vi "Modules - Explorer.vi"(8 "error in":errorcluster) -> (0 "error out":errorcluster)   [LabVIEW 2019]
uses:
  Controls/Explorer - State.ctl
  Controls/eFGV States.ctl
  Controls/Explorer - Data Structure.ctl
  <vilib>/httpClient/ClientHandle.ctl
  Controls/FGV States.ctl
  Controls/JSON - Fileid.ctl
  <vilib>/httpClient/POSTBuffer.vi
  <vilib>/httpClient/LabVIEWHTTPClient.lvlib
panel:
  in  "Pin":bool
  in  "Refresh":bool
  in  "Tab":enum32{"Running", "Archive"}(radio)
  in  "TreeDone":string(tree)
  in  "TreeRun":string(tree)
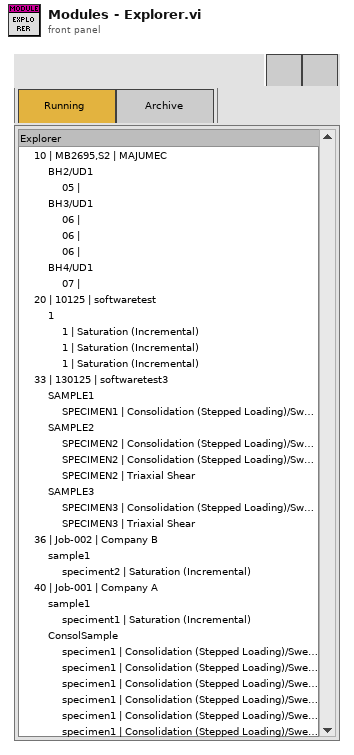
[diagram p1: front panel]
types:
  T1 = typedef "Explorer - State.ctl" = enum16{"Init", "Idle", "DoubleClick", "GetInfo", "Porpulate", "Sort", "Prepare to Load", "Load", "Close", "Exit"}
  T2 = enum32{"invalid app kind", "Development System", "Run Time System", "Student Edition", "Embedded LabVIEW", "Evaluation", "Custom"}
  T3 = typedef "Explorer - Data Structure.ctl" = cluster{"Ref":T4, "TestData":string, "TestNameRun":string[], "TestNameDone":string[], "Selected Tag":string, "Selected Index":i32, "LoadRun?":bool, "NameRun":string[], "NameDone":string[], "fileid":string[], "testname":string[]}
  T4 = typedef "LabVIEWHTTPClient.lvlib/ClientHandle.ctl" = refnum<k1>
  T5 = typedef "eFGV States.ctl" = enum16{"Init", "Read", "Write", "Exit"}
  T6 = enum32{"Invalid", "Standard", "Closed", "Hidden", "Minimized", "Maximized"}
  T7 = typedef "FGV States.ctl" = enum16{"Read", "Write"}
  T8 = typedef "JSON - Fileid.ctl" = cluster{"status":string, "data":cluster{"id":string, "created_date":string, "testname":string, "jobno":string, "jobdesc":string, "sampleid":string, "date":string, "specimentno":string, "depth":string, "height":string, "diameter":string, "weight":string, "done":string}[]}
  T9 = cluster{"RunTest":refnum<vi>, "Name":string, "FileId":string, "Status":string}
  T10 = cluster{"id":string, "created_date":string, "testname":string, "jobno":string, "jobdesc":string, "sampleid":string, "date":string, "specimentno":string, "depth":string, "height":string, "diameter":string, "weight":string, "done":string}[]
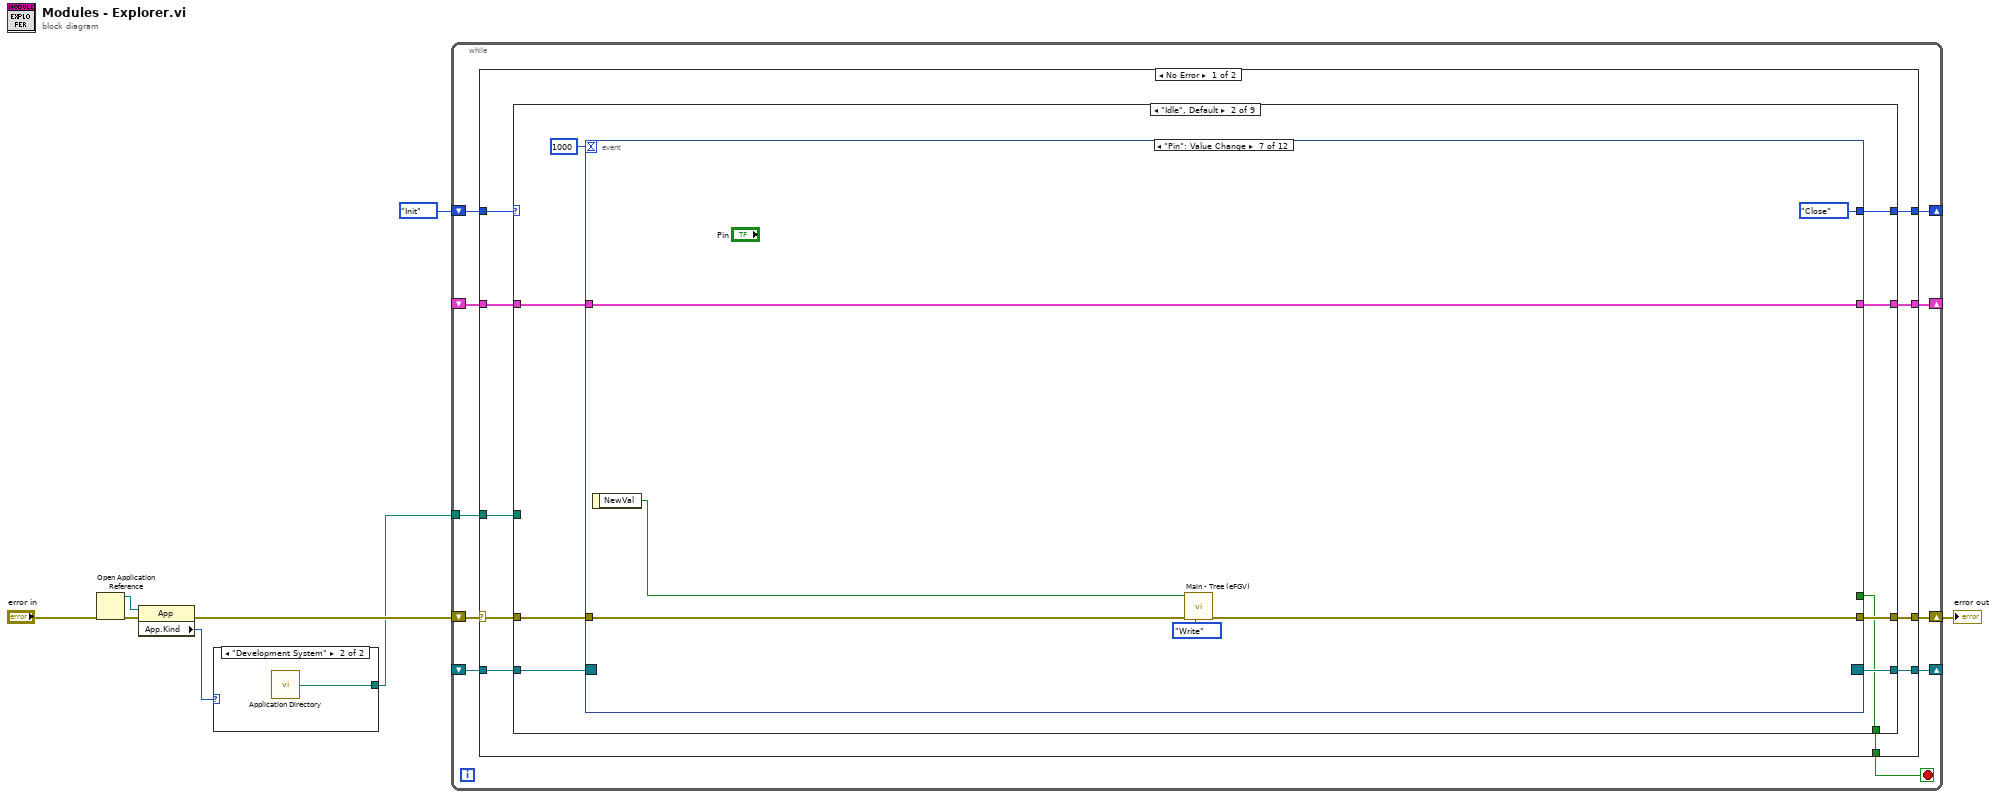
[diagram p0: block diagram]
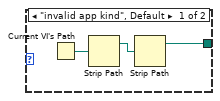
[diagram p2: hidden frame]
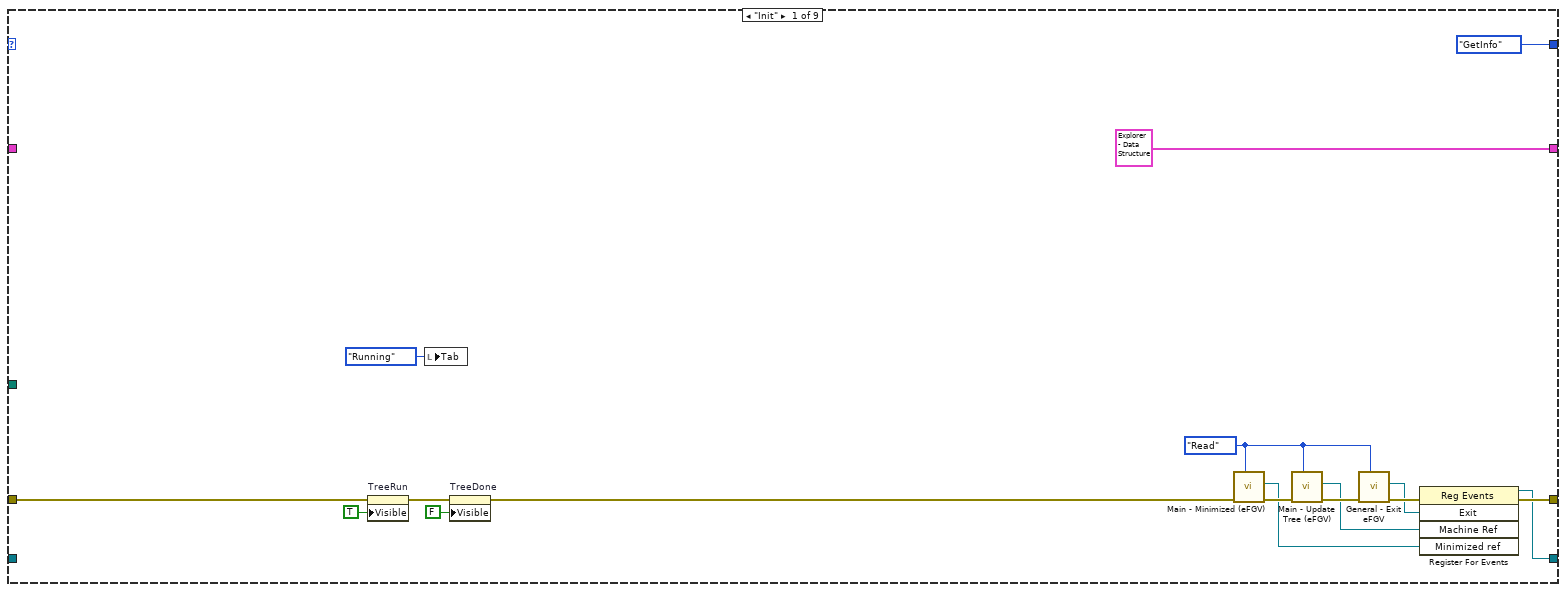
[diagram p3: hidden frame]
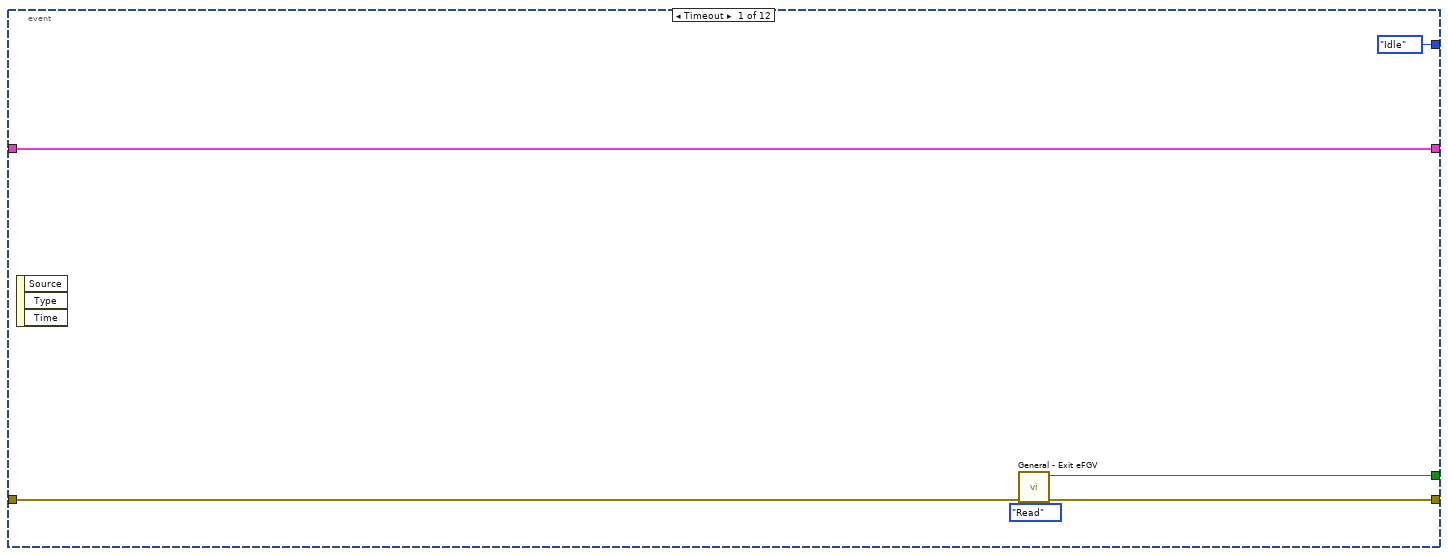
[diagram p4: hidden frame]
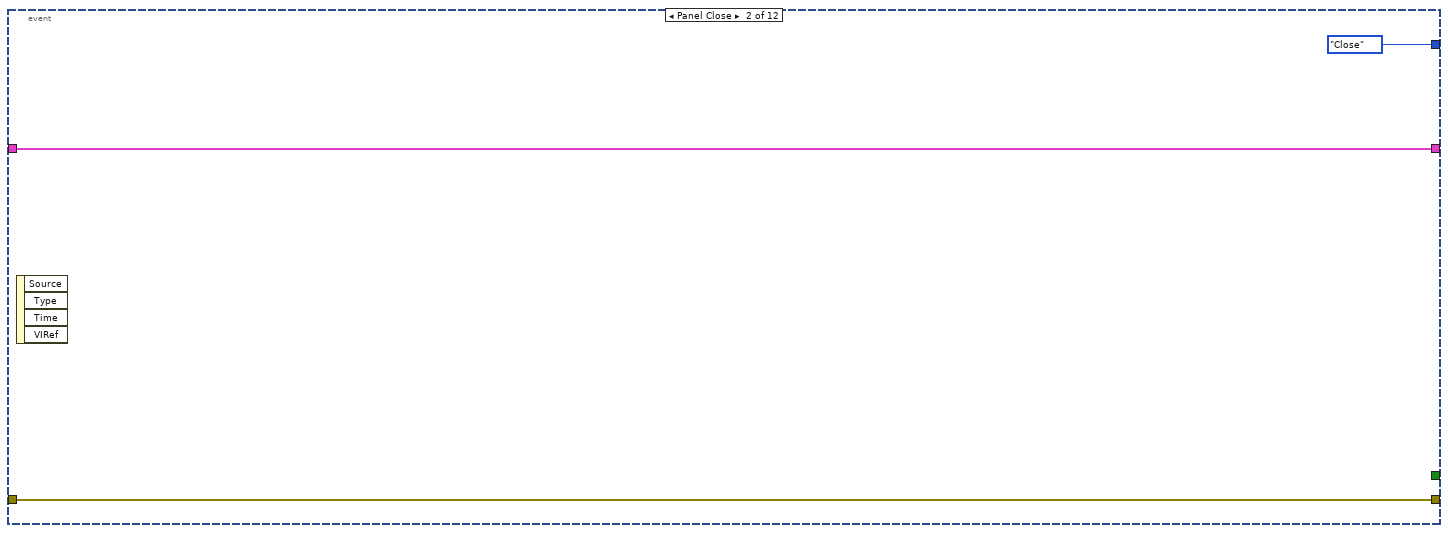
[diagram p5: hidden frame]
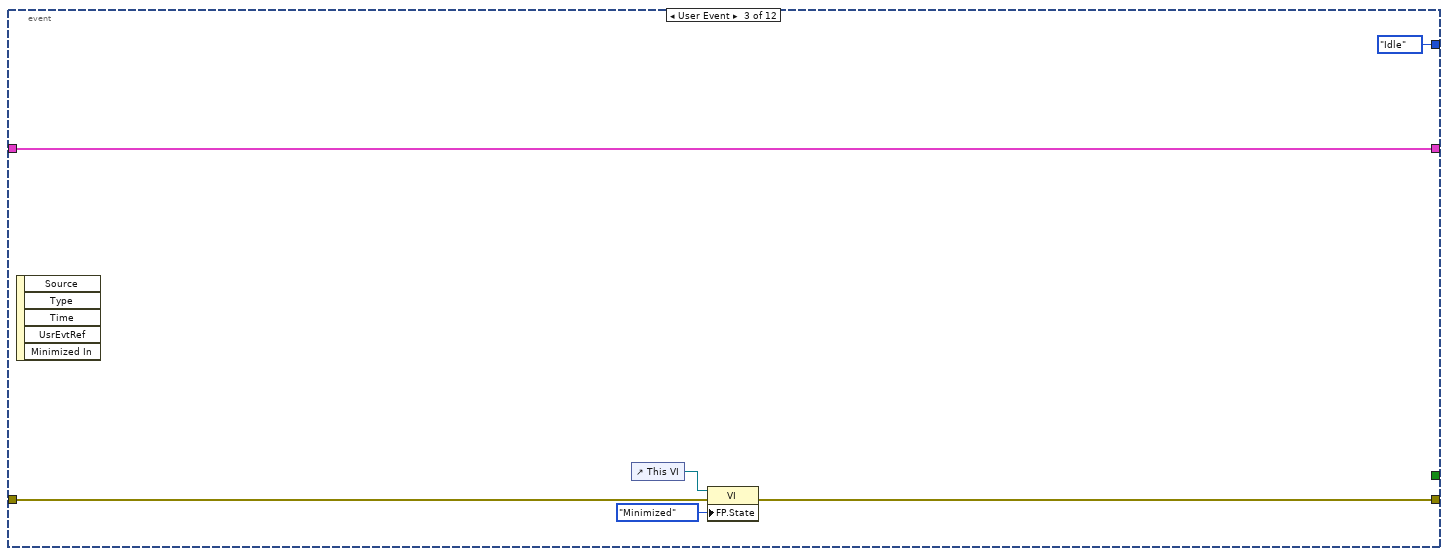
[diagram p6: hidden frame]
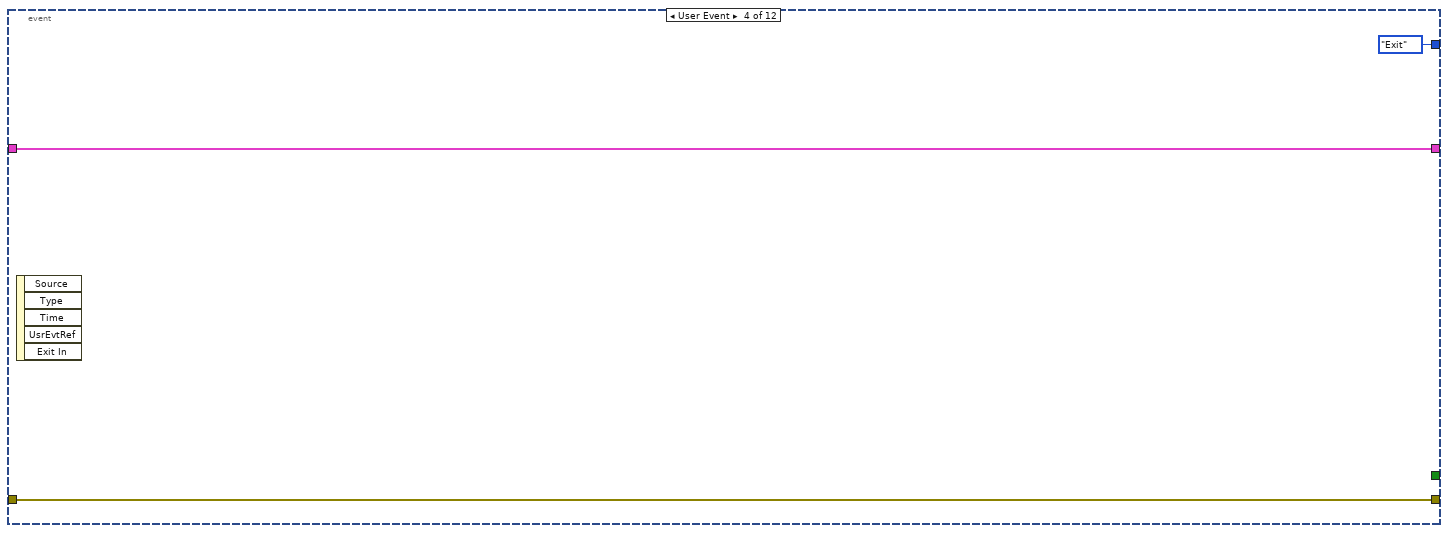
[diagram p7: hidden frame]
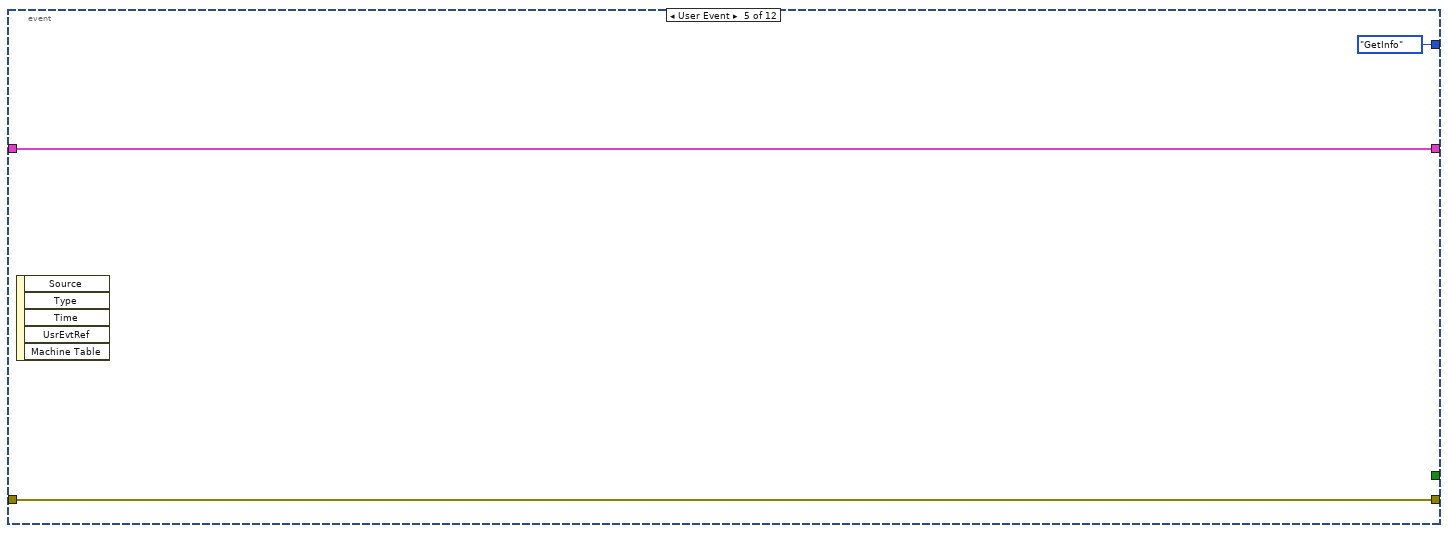
[diagram p8: hidden frame]
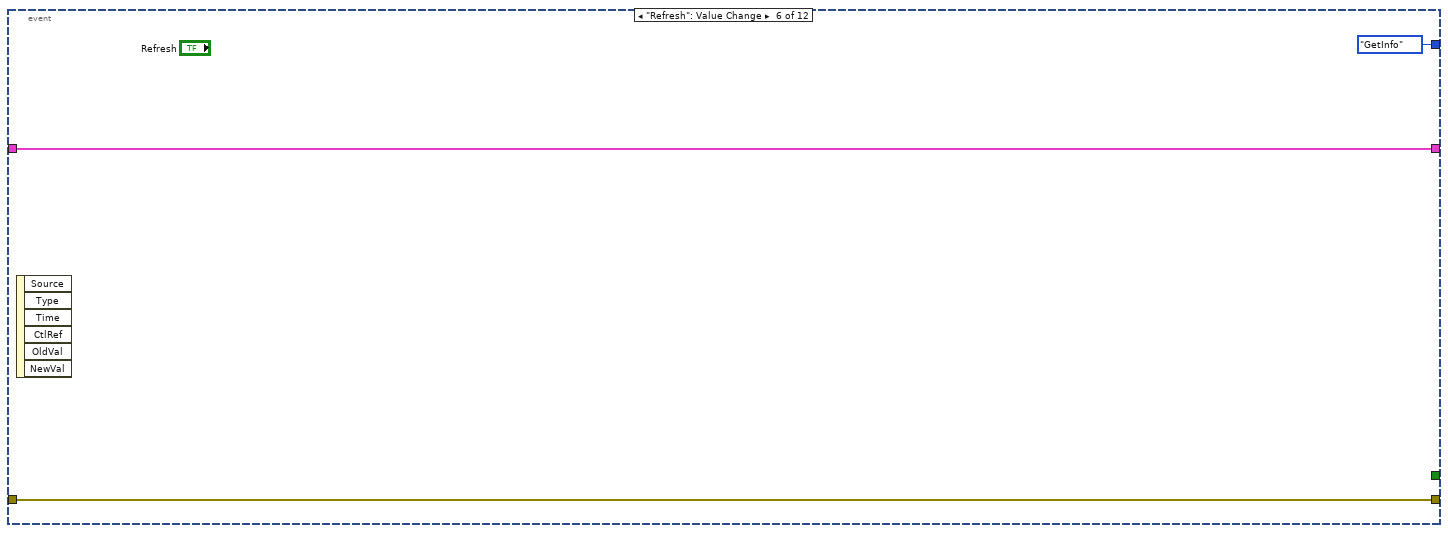
[diagram p9: hidden frame]
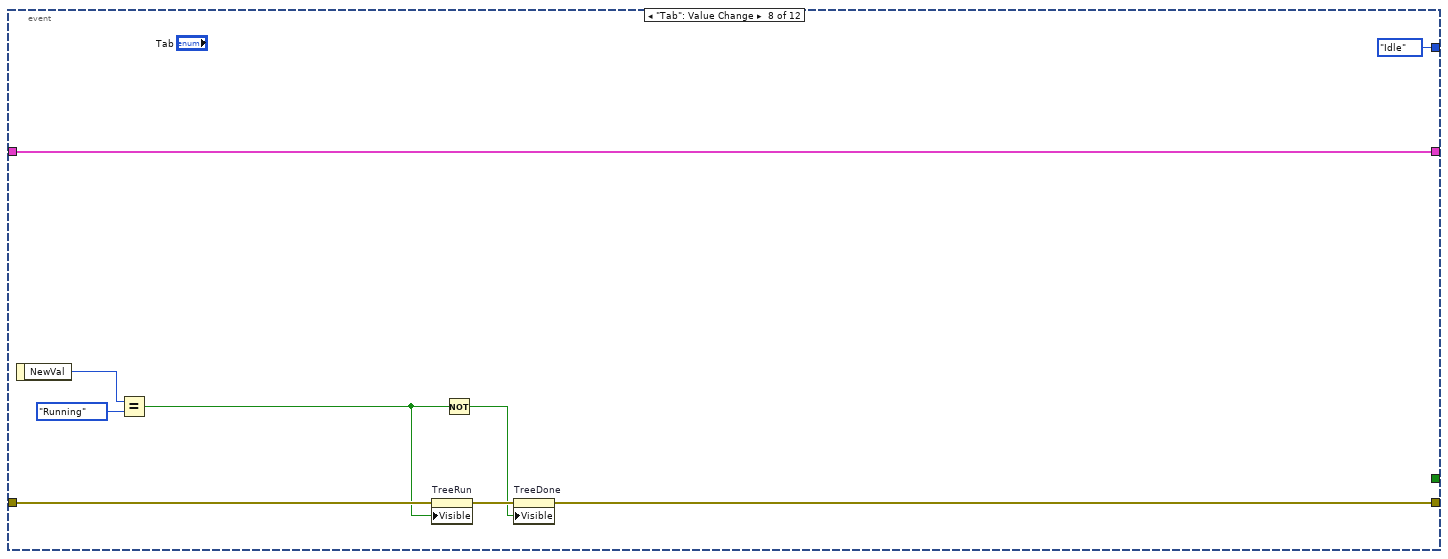
[diagram p10: hidden frame]
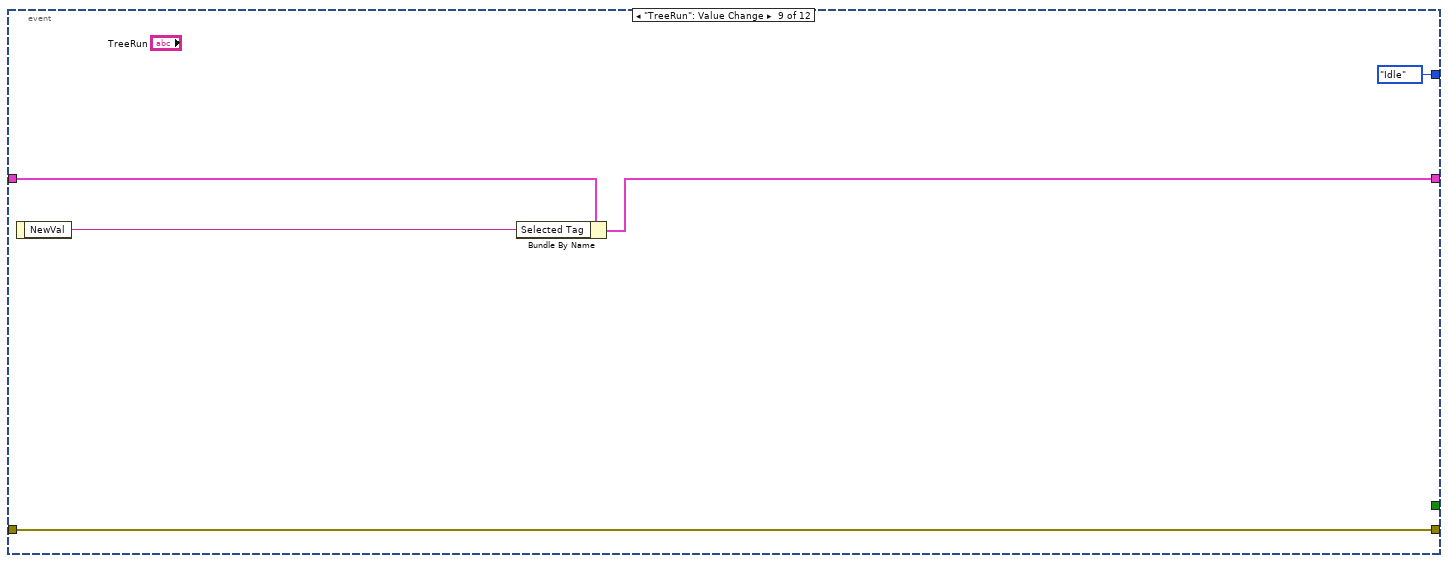
[diagram p11: hidden frame]
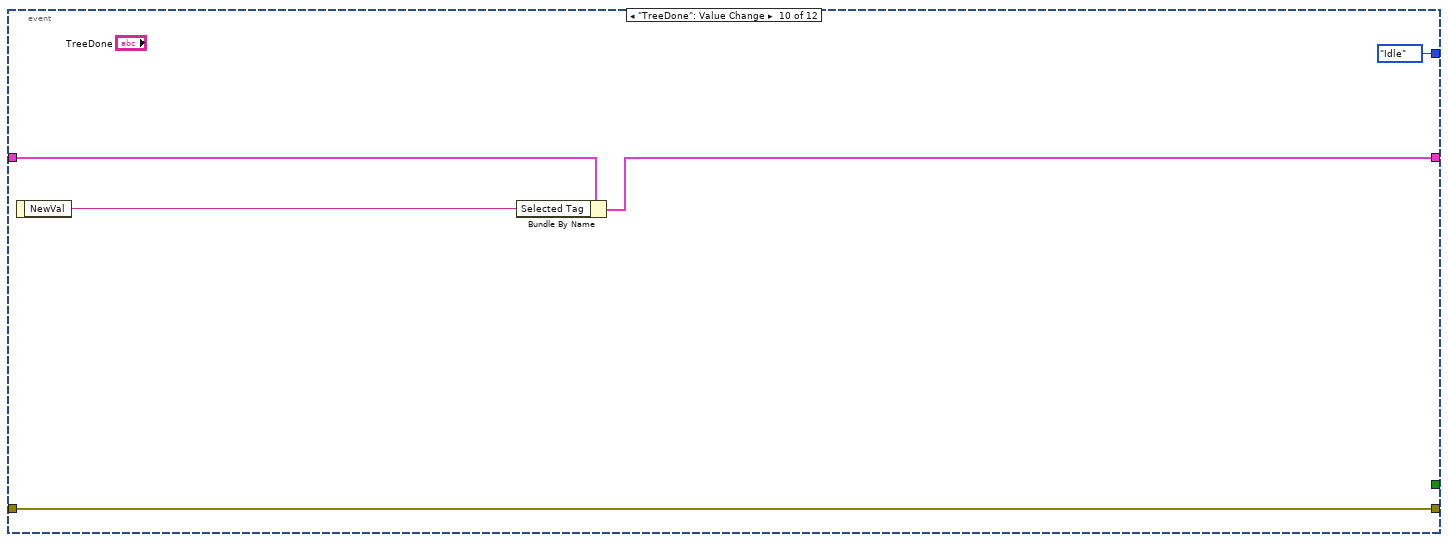
[diagram p12: hidden frame]
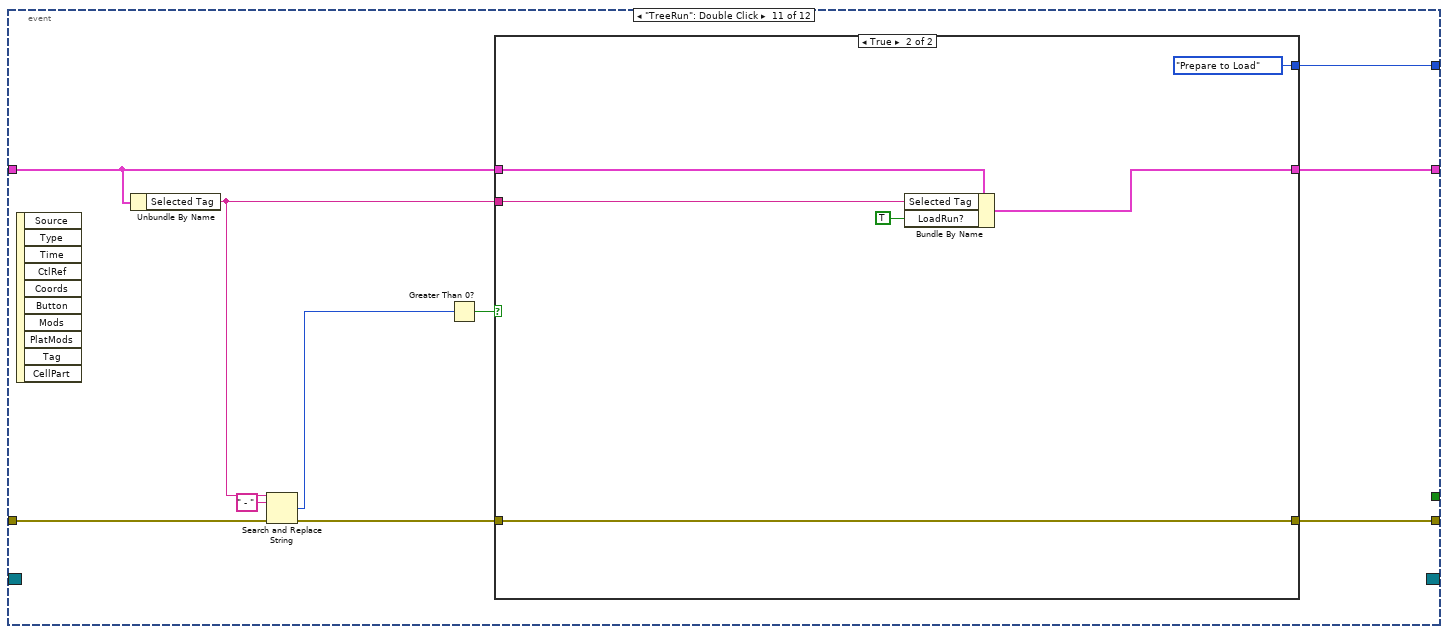
[diagram p13: hidden frame]
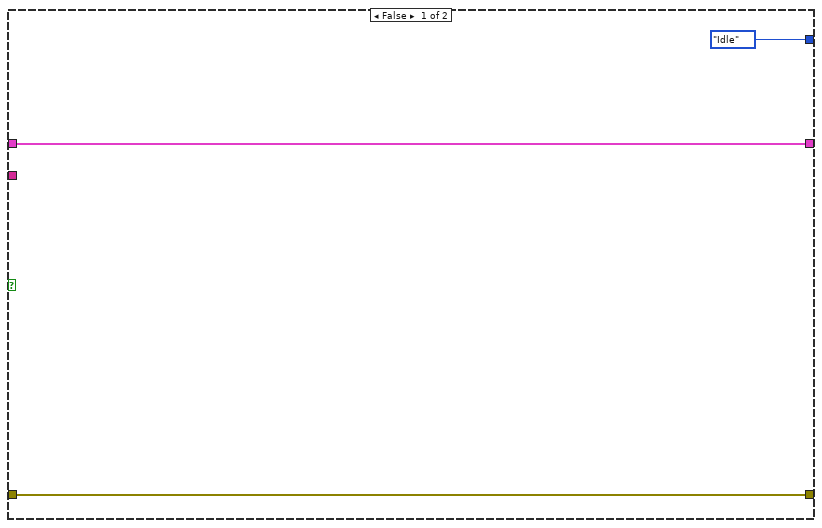
[diagram p14: hidden frame]
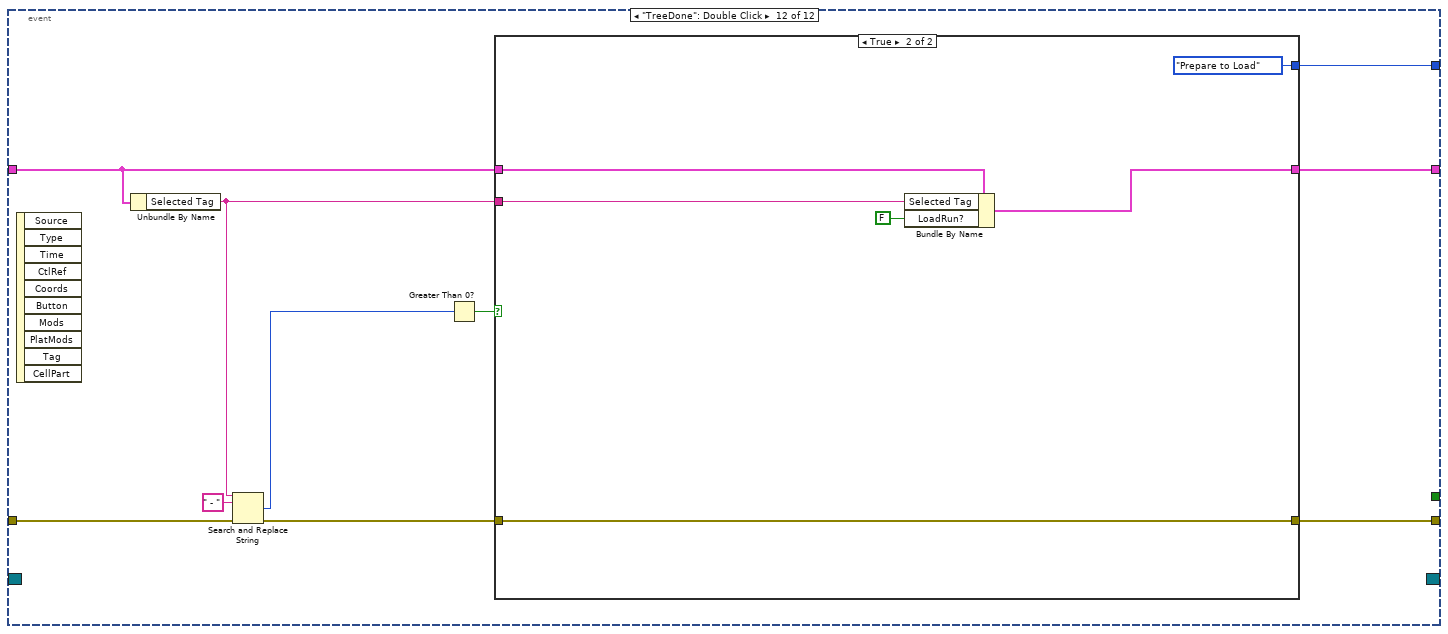
[diagram p15: hidden frame]
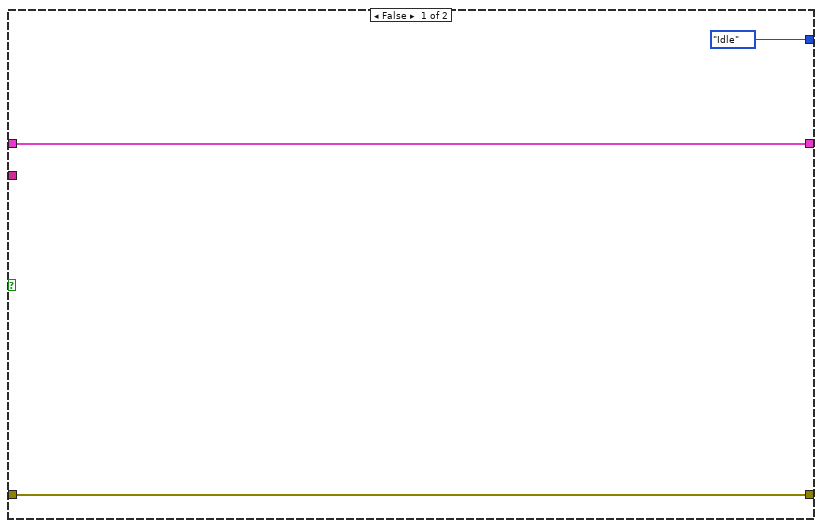
[diagram p16: hidden frame]
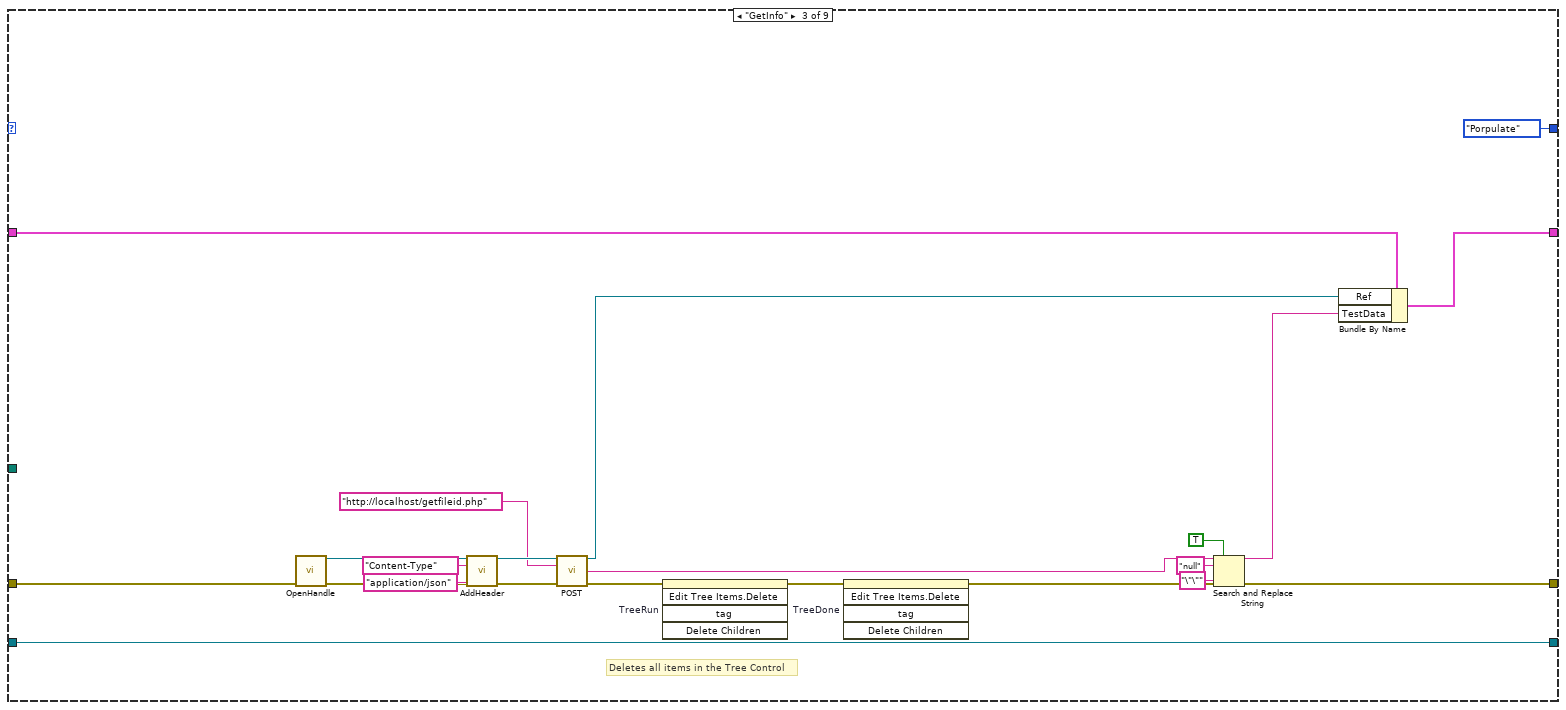
[diagram p17: hidden frame]
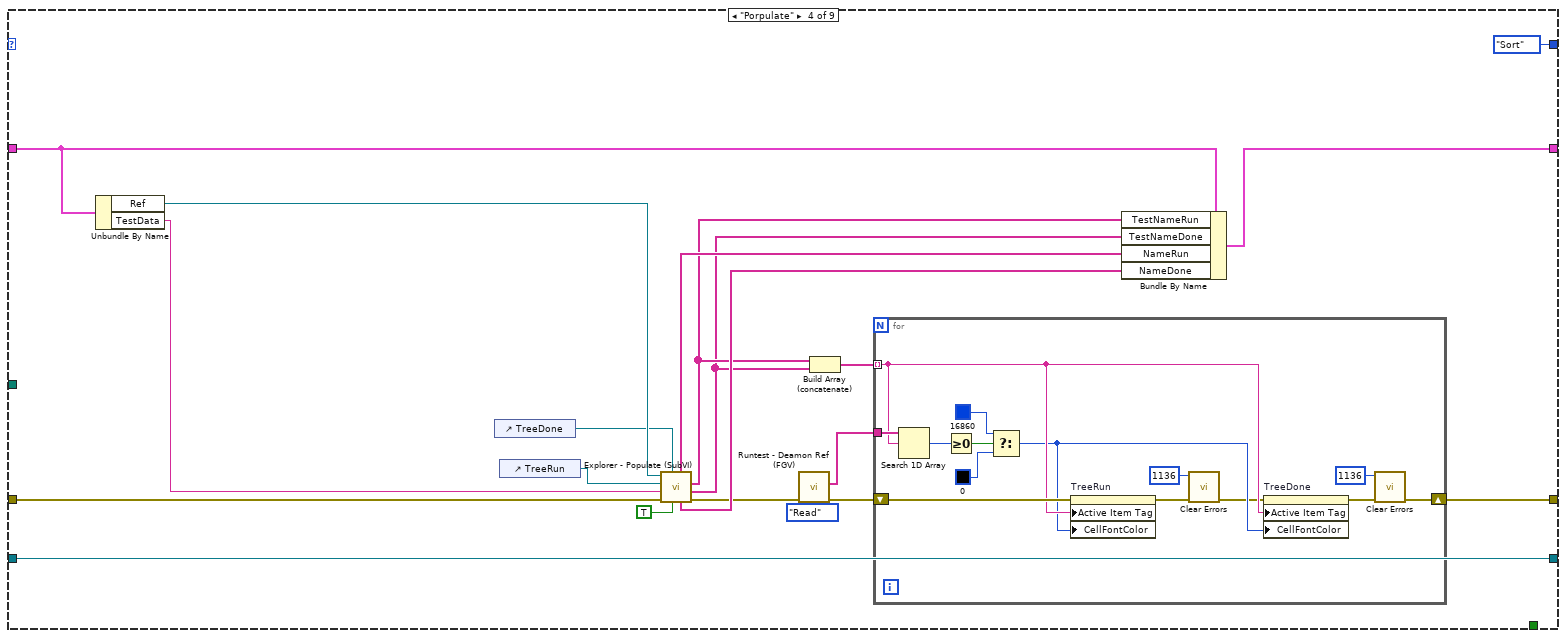
[diagram p18: hidden frame]
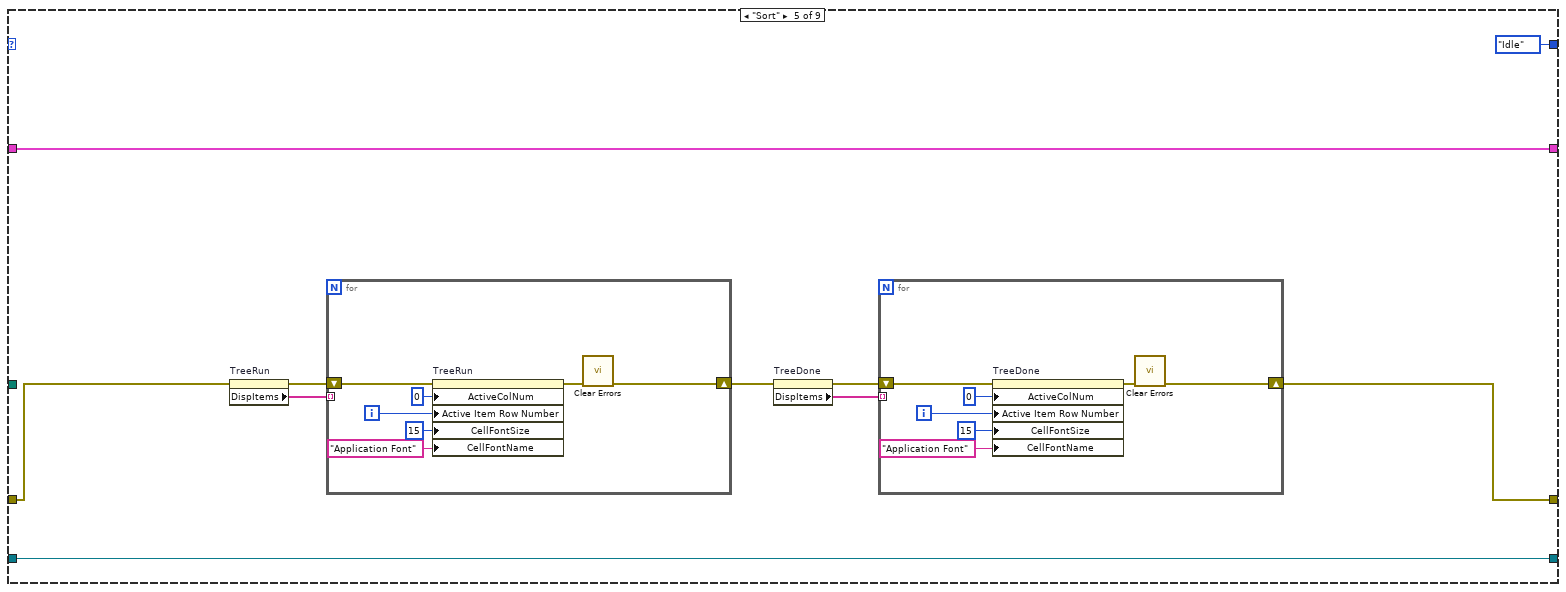
[diagram p19: hidden frame]
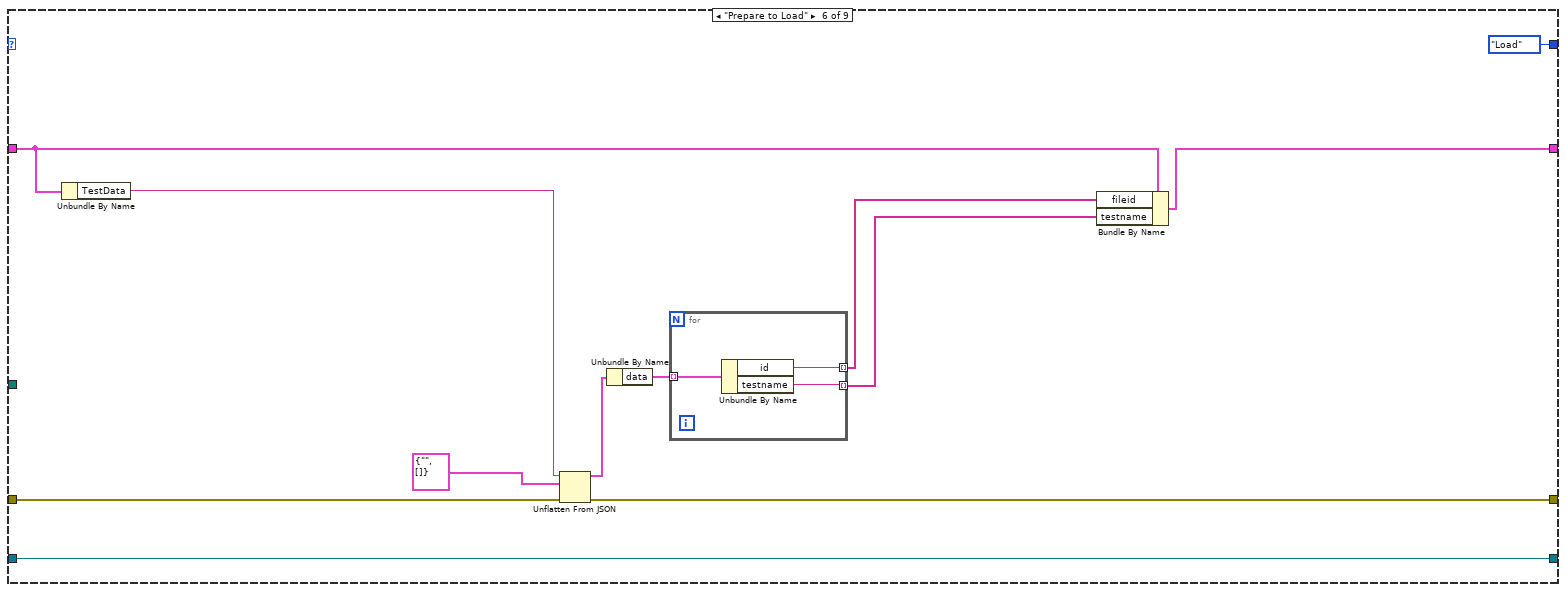
[diagram p20: hidden frame]
diagram:
  n1 = Open Application Reference(8:"error in") -> (0:w6:errorcluster, 3:w5:refnum<vi>)  [unwired: 3 in]
  n2 = property class="App"(reference=w5, error in=w6) -> (error out=w2:errorcluster, "App.Kind"=w4:T2)  [unwired: 1 out]
  n3 = case shown="\"Development System\"" w4 {
    tunnel: [w9 w12] -> w1
    frame "invalid app kind", Default {
      n4 = Current VI's Path() -> (path=w11:path)
      n5 = Strip Path(path=w11) -> (stripped path=w10:path)  [unwired: 1 out]
      n6 = Strip Path(path=w10) -> (stripped path=w9:path)  [unwired: 1 out]
    }
    frame "Development System" {
      n7 = call <vilib>:"Application Directory.vi"() -> ("Application Directory"=w12:path)
    }
  }
  n8 = while {
    shift-right: [w21] -> w8
    shift-left: w2 -> [w22]
    shift-right: [w19] -> _
    shift-left: _ -> [w18]
    shift-right: [w16] -> _
    shift-left: Explorer_-_State."Init" ("Enum") -> [w17]
    shift-right: [w15] -> _
    shift-left: _ -> [w14]
    tunnel: w1 -> [w13]
    stop <- w20 stop-if-true
    n9 = case shown="No Error" w22 {
      selector: w22 -> [w32 w433]
      tunnel: [w31 w432] -> w21
      tunnel: [w30 _] -> w20
      tunnel: [w29 w430] -> w19
      tunnel: w18 -> [w28 w430]
      tunnel: w17 -> [w27 _]
      tunnel: [w26 Explorer_-_State."Idle" ("Enum")] -> w16
      tunnel: [w25 w429] -> w15
      tunnel: w14 -> [w24 w429]
      tunnel: w13 -> [w23 _]
      frame No Error {
        n10 = case shown="\"Idle\", Default" w27 {
          tunnel: w32 -> [w38 w57 w151 w185 w207 w234 w246 w418 w426]
          tunnel: [w47 w58 w150 w168 w202 w235 w247 w417 w426] -> w31
          tunnel: [_ w50 _ _ _ _ _ _ TRUE] -> w30
          tunnel: [w46 w55 w167 w187 w211 w237 w248 w422 w423] -> w29
          tunnel: w28 -> [_ w56 w167 w187 w211 w237 w248 w422 w423]
          tunnel: [Explorer_-_State."GetInfo" ("Enum") w54 Explorer_-_State."Porpulate" ("Enum") Explorer_-_State."Sort" ("Enum") Explorer_-_State."Idle" ("Enum") Explorer_-_State."Load" ("Enum") Explorer_-_State."Idle" ("Enum") Explorer_-_State."Idle" ("Enum") Explorer_-_State."Exit" ("Enum")] -> w26
          tunnel: [T3 {"Ref"=refnum, "TestData"="", "TestNameRun"=[], "TestNameDone"=[], "Selected Tag"="", "Selected Index"=0, "LoadRun?"=FALSE, "NameRun"=[], "NameDone"=[], "fileid"=[], "testname"=[]} w53 w149 w181 w208 w227 w243 w421 w424] -> w25
          tunnel: w24 -> [_ w52 w148 w180 w208 w226 w242 w421 w424]
          tunnel: w23 -> [_ _ _ _ _ _ w241 _ _]
          frame "Init" {
            w33 = eFGV_States."Read" ("eFGV States")
            n11 = property on="TreeRun" class="Tree (strict)"(error in=w38, "Visible"=TRUE) -> (error out=w39:errorcluster)  [unwired: 1 in, 1 out]
            n12 = local write "Tab"(enum32{"Running", "Archive"}."Running" ("Tab")) -> ()
            n13 = property on="TreeDone" class="Tree (strict)"(error in=w39, "Visible"=FALSE) -> (error out=w36:errorcluster)  [unwired: 1 in, 1 out]
            n14 = call "Main - Minimized (eFGV).vi"("Action"=w33, "error in"=w36) -> ("error out"=w35:errorcluster, "Minimized ref"=w34:refnum<user-event>)  [unwired: 7 in, 1 out]
            n15 = call "Main - Update Tree (eFGV).vi"("Action"=w33, "error in"=w35) -> ("error out"=w43:errorcluster, "Machine Ref"=w42:refnum<user-event>)  [unwired: 7 in, 1 out]
            n16 = call "General - Exit eFGV.vi"("eFGV States"=w33, "error in (no error)"=w43) -> ("error out"=w49:errorcluster, "Exit"=w48:refnum<user-event>)  [unwired: 7 in, 1 out]
            n17 = register-events(error in=w49, w48, w42, w34) -> (reference out=w46:refnum<event-registration>, error out=w47:errorcluster)  [unwired: 1 in]
          }
          frame "Idle", Default {
            n18 = event shown="[6] \"Pin\": Value Change" {
              selector: w56 -> [_ _ _ _ _ _ _ _ _ _ _ _]
              dyn-events: [_ _ _ _ _ _ _ _ _ _ _ _] -> w55
              timeout: 1000 -> [_ _ _ _ _ _ _ _ _ _ _ _]
              tunnel: w57 -> [w60 w67 w68 w76 w79 w82 w85 w93 w101 w106 w111 w130]
              tunnel: [w61 w67 w69 w76 w79 w82 w86 w94 w101 w106 w116 w135] -> w58
              tunnel: [Explorer_-_State."Idle" ("Enum") Explorer_-_State."Close" ("Enum") Explorer_-_State."Idle" ("Enum") Explorer_-_State."Exit" ("Enum") Explorer_-_State."GetInfo" ("Enum") Explorer_-_State."GetInfo" ("Enum") Explorer_-_State."Close" ("Enum") Explorer_-_State."Idle" ("Enum") Explorer_-_State."Idle" ("Enum") Explorer_-_State."Idle" ("Enum") w113 w132] -> w54
              tunnel: [w63 w65 w73 w75 w78 w81 w88 w97 w100 w105 w114 w133] -> w53
              tunnel: w52 -> [w63 w65 w73 w75 w78 w81 w88 w97 w99 w104 w115 w134]
              tunnel: [w59 _ _ _ _ _ _ _ _ _ _ _] -> w50
              event Timeout {
                n19 = event-data() -> ()  [unwired: 1 in, 3 out]
                n20 = call "General - Exit eFGV.vi"("eFGV States"=eFGV_States."Read", "error in (no error)"=w60) -> ("error out"=w61:errorcluster, "Exit Out"=w59:bool)  [unwired: 7 in, 1 out]
              }
              event Panel Close {
                n21 = event-data() -> ()  [unwired: 1 in, 4 out]
              }
              event User Event {
                n22 = event-data() -> ()  [unwired: 1 in, 5 out]
                n23 = control-ref of="This VI"() -> (w71:refnum<vi>)
                n24 = property class="VI"(reference=w71, error in=w68, "FP.State"=T6."Minimized" ("Front Panel Window:State")) -> (error out=w69:errorcluster)  [unwired: 1 out]
              }
              event User Event {
                n25 = event-data() -> ()  [unwired: 1 in, 5 out]
              }
              event User Event {
                n26 = event-data() -> ()  [unwired: 1 in, 5 out]
              }
              event "Refresh": Value Change {
                n27 = event-data() -> ()  [unwired: 1 in, 6 out]
              }
              event "Pin": Value Change {
                n28 = event-data() -> ("NewVal"=w84:bool)  [unwired: 1 in]
                n29 = call "Main - Tree (eFGV).vi"("Action"=eFGV_States."Write", "error in"=w85, "Pin"=w84) -> ("error out"=w86:errorcluster)  [unwired: 6 in, 2 out]
              }
              event "Tab": Value Change {
                n30 = event-data() -> ("NewVal"=w92:enum32{"Running", "Archive"})  [unwired: 1 in]
                n31 = Equal?(x=w92, y=enum32{"Running", "Archive"}."Running") -> (x = y?=w90:bool)
                n32 = property on="TreeRun" class="Tree (strict)"(error in=w93, "Visible"=w90) -> (error out=w95:errorcluster)  [unwired: 1 in, 1 out]
                n33 = Not(x=w90) -> (.not. x?=w89:bool)
                n34 = property on="TreeDone" class="Tree (strict)"(error in=w95, "Visible"=w89) -> (error out=w94:errorcluster)  [unwired: 1 in, 1 out]
              }
              event "TreeRun": Value Change {
                n35 = event-data() -> ("NewVal"=w98:string)  [unwired: 1 in]
                n36 = Bundle By Name(cluster=w99, "Selected Tag"=w98) -> (w100:T3)
              }
              event "TreeDone": Value Change {
                n37 = event-data() -> ("NewVal"=w103:string)  [unwired: 1 in]
                n38 = Bundle By Name(cluster=w104, "Selected Tag"=w103) -> (w105:T3)
              }
              event "TreeRun": Double Click {
                n39 = event-data() -> ()  [unwired: 1 in, 10 out]
                n40 = Unbundle By Name(w115) -> ("Selected Tag"=w110:string)
                n41 = Search and Replace String(input string=w110, search string=" - ", error in=w111) -> (number of replacements=w108:i32, error out=w112:errorcluster)  [unwired: 5 in, 2 out]
                n42 = Greater Than 0?(x=w108) -> (x > 0?=w117:bool)
                n43 = case shown="True" w117 {
                  tunnel: w112 -> [w120 w122]
                  tunnel: [w120 w122] -> w116
                  tunnel: w115 -> [w119 w126]
                  tunnel: [w119 w125] -> w114
                  tunnel: w110 -> [_ w121]
                  tunnel: [Explorer_-_State."Idle" ("Enum") Explorer_-_State."Prepare to Load" ("Enum")] -> w113
                  frame False {
                  }
                  frame True {
                    n44 = Bundle By Name(cluster=w126, "Selected Tag"=w121, "LoadRun?"=TRUE) -> (w125:T3)
                  }
                }
              }
              event "TreeDone": Double Click {
                n45 = event-data() -> ()  [unwired: 1 in, 10 out]
                n46 = Unbundle By Name(w134) -> ("Selected Tag"=w129:string)
                n47 = Search and Replace String(input string=w129, search string=" - ", error in=w130) -> (number of replacements=w127:i32, error out=w131:errorcluster)  [unwired: 5 in, 2 out]
                n48 = Greater Than 0?(x=w127) -> (x > 0?=w136:bool)
                n49 = case shown="True" w136 {
                  tunnel: w131 -> [w139 w141]
                  tunnel: [w139 w141] -> w135
                  tunnel: w134 -> [w138 w145]
                  tunnel: [w138 w144] -> w133
                  tunnel: w129 -> [_ w140]
                  tunnel: [Explorer_-_State."Idle" ("Enum") Explorer_-_State."Prepare to Load" ("Enum")] -> w132
                  frame False {
                  }
                  frame True {
                    n50 = Bundle By Name(cluster=w145, "Selected Tag"=w140, "LoadRun?"=FALSE) -> (w144:T3)
                  }
                }
              }
            }
          }
          frame "GetInfo" {
            # "Deletes all items in the Tree Control"
            n51 = call <vilib>:"OpenHandle.vi"("error in (no error)"=w151) -> ("client handle out"=w162:T4, "error out"=w160:errorcluster)  [unwired: 13 in]
            n52 = call <vilib>:"AddHeader.vi"("client handle"=w162, "header"="Content-Type", "value"="application/json", "error in (no error)"=w160) -> ("client handle out"=w163:T4, "error out"=w161:errorcluster)  [unwired: 10 in]
            n53 = call-poly <vilib>:"POST.vi"("client handle"=w163, "url"="http://localhost/getfileid.php", "error in (no error)"=w161) -> ("client handle out"=w153:T4, "body"=w156:string, "error out"=w158:errorcluster)  [unwired: 9 in, 1 out]
            n54 = invoke on="TreeRun" class="Tree (strict)" method="Edit Tree Items.Delete"(error in=w158) -> (error out=w147:errorcluster)  [unwired: 4 in, 4 out]
            n55 = invoke on="TreeDone" class="Tree (strict)" method="Edit Tree Items.Delete"(error in=w147) -> (error out=w146:errorcluster)  [unwired: 4 in, 4 out]
            n56 = Search and Replace String(replace all?=TRUE ("replace all? (F)"), input string=w156, search string="null", replace string="\"\"" ("replace string (\"\")"), error in=w146) -> (result string=w152:string, error out=w150:errorcluster)  [unwired: 3 in, 2 out]
            n57 = Bundle By Name(cluster=w148, "Ref"=w153, "TestData"=w152) -> (w149:T3)
          }
          frame "Porpulate" {
            n58 = Unbundle By Name(w180) -> ("Ref"=w183:T4, "TestData"=w184:string)
            n59 = control-ref of="TreeDone"() -> (w179:refnum<vi>)
            n60 = control-ref of="TreeRun"() -> (w182:refnum<vi>)
            n61 = call "Explorer - Populate (SubVI).vi"("Asc?"=TRUE, "TreeDone"=w179, "error in (no error)"=w185, "Test Data"=w184, "TreeRun"=w182, "RefIn"=w183) -> ("error out"=w174:errorcluster, "TestName Done"=w171:string[], "TestName Running"=w172:string[], "Name Done"=w176:string[], "Name Running"=w177:string[])  [unwired: 1 out]
            n62 = call "Runtest - Deamon Ref (FGV).vi"("Action"=FGV_States."Read", "error in"=w174) -> ("error out"=w169:errorcluster, "Name out"=w173:string[])  [unwired: 7 in, 1 out]
            n63 = Build Array (concatenate)(w172, w171) -> (w170:string[])
            n64 = for {
              tunnel: w173 -> [w201]
              tunnel: w170 -> [w193] mode=indexing
              shift-right: [w189] -> w168
              shift-left: w169 -> [w196]
              n65 = Search 1D Array(1D array=w201, element=w193) -> (index of element=w200:i32)  [unwired: 1 in]
              n66 = Greater Or Equal To 0?(x=w200) -> (x >= 0?=w199:bool)
              n67 = Select(t=u32 16860 ("Active Cell:Cell Font:Color"), s=w199, f=u32 0 ("Active Cell:Cell Font:Color")) -> (s? t:f=w192:u32)
              n68 = property on="TreeRun" class="Tree (strict)"(error in=w196, "Active Item Tag"=w193, "CellFontColor"=w192) -> (error out=w195:errorcluster)  [unwired: 1 in, 1 out]
              n69 = call <vilib>:"Clear Errors.vi"("error in (no error)"=w195, "specific error code to clear (0: all)"=1136) -> ("error out"=w191:errorcluster)  [unwired: 4 in, 1 out]
              n70 = property on="TreeDone" class="Tree (strict)"(error in=w191, "Active Item Tag"=w193, "CellFontColor"=w192) -> (error out=w194:errorcluster)  [unwired: 1 in, 1 out]
              n71 = call <vilib>:"Clear Errors.vi"("error in (no error)"=w194, "specific error code to clear (0: all)"=1136) -> ("error out"=w189:errorcluster)  [unwired: 4 in, 1 out]
            }
            n72 = Bundle By Name(cluster=w180, "TestNameRun"=w172, "TestNameDone"=w171, "NameRun"=w177, "NameDone"=w176) -> (w181:T3)
          }
          frame "Sort" {
            n73 = property on="TreeRun" class="Tree (strict)"(error in=w207) -> (error out=w209:errorcluster, "DispItems"=w206:string[])  [unwired: 1 in, 1 out]
            n74 = for {
              shift-right: [w219] -> w205
              shift-left: w209 -> [w225]
              tunnel: w206 -> [_] mode=indexing
              i -> [w222]
              n75 = property on="TreeRun" class="Tree (strict)"(error in=w225, "ActiveColNum"=0 ("Active Item:Row Number"), "Active Item Row Number"=w222, "CellFontSize"=u32 15 ("Active Cell:Cell Font:Size"), "CellFontName"="Application Font" ("Active Cell:Cell Font:Name")) -> (error out=w220:errorcluster)  [unwired: 1 in, 1 out]
              n76 = call <vilib>:"Clear Errors.vi"("error in (no error)"=w220) -> ("error out"=w219:errorcluster)  [unwired: 5 in, 1 out]
            }
            n77 = property on="TreeDone" class="Tree (strict)"(error in=w205) -> (error out=w204:errorcluster, "DispItems"=w203:string[])  [unwired: 1 in, 1 out]
            n78 = for {
              shift-right: [w218] -> w202
              shift-left: w204 -> [w217]
              tunnel: w203 -> [_] mode=indexing
              i -> [w214]
              n79 = property on="TreeDone" class="Tree (strict)"(error in=w217, "ActiveColNum"=0 ("Active Item:Row Number"), "Active Item Row Number"=w214, "CellFontSize"=u32 15 ("Active Cell:Cell Font:Size"), "CellFontName"="Application Font" ("Active Cell:Cell Font:Name")) -> (error out=w216:errorcluster)  [unwired: 1 in, 1 out]
              n80 = call <vilib>:"Clear Errors.vi"("error in (no error)"=w216) -> ("error out"=w218:errorcluster)  [unwired: 5 in, 1 out]
            }
          }
          frame "Prepare to Load" {
            n81 = Unbundle By Name(w226) -> ("TestData"=w233:string)
            n82 = Unflatten From JSON(JSON string=w233, type and defaults=T8 {"status"="", "data"=[]}, error in (no error)=w234) -> (value=w232:T8, error out=w235:errorcluster)  [unwired: 4 in]
            n83 = Unbundle By Name(w232) -> ("data"=w230:T10)
            n84 = for {
              tunnel: w230 -> [w240] mode=indexing
              tunnel: [w239] -> w229 mode=indexing
              tunnel: [w238] -> w228 mode=indexing
              n85 = Unbundle By Name(w240) -> ("id"=w239:string, "testname"=w238:string)
            }
            n86 = Bundle By Name(cluster=w226, "fileid"=w229, "testname"=w228) -> (w227:T3)
          }
          frame "Load" {
            n87 = Unbundle By Name(w242) -> ("LoadRun?"=w244:bool)
            n88 = case shown="True" w244 {
              tunnel: [w268 w352] -> w247
              tunnel: w246 -> [w263 w347]
              tunnel: [w271 w356] -> w243
              tunnel: w242 -> [w271 w356]
              tunnel: w241 -> [w266 w350]
              frame False {
                (unwired) "Modules - Run Test with Config Load.vit"
                n89 = Unbundle By Name(w271) -> ("testname"=w253:string[], "Selected Tag"=w252:string, "NameDone"=w257:string[], "TestNameDone"=w258:string[], "fileid"=w251:string[])
                n90 = Build Path(base path=w266, name or relative path="Modules") -> (appended path=w270:path)
                n91 = Search 1D Array(1D array=w258, element=w252) -> (index of element=w259:i32)  [unwired: 1 in]
                n92 = Build Path(base path=w270, name or relative path="Modules - Run Test with Config Load - ausie.vit") -> (appended path=w267:path)
                n93 = Match Pattern(string=w252, regular expression="_") -> (before substring=w254:string)  [unwired: 1 in, 3 out]
                n94 = call "Runtest - Deamon Ref (FGV).vi"("Action"=FGV_States."Read", "error in"=w263) -> ("error out"=w264:errorcluster, "Name out"=w260:string[], "Ref out"=w261:refnum<vi>[])  [unwired: 7 in]
                n95 = Index Array(array=w257, index=w259) -> (element=w256:string)
                n96 = Search 1D Array(1D array=w253, element=w254) -> (index of element=w250:i32)  [unwired: 1 in]
                n97 = Search 1D Array(1D array=w260, element=w252) -> (index of element=w262:i32)  [unwired: 1 in]
                n98 = case shown="-1" w262 {
                  selector: w262 -> [w277 _]
                  tunnel: [w279 w306] -> w268
                  tunnel: w267 -> [_ w310]
                  tunnel: w264 -> [w280 w309]
                  tunnel: w252 -> [_ w301]
                  tunnel: w261 -> [w278 w305]
                  tunnel: w260 -> [_ w302]
                  tunnel: w256 -> [w275 w299]
                  tunnel: w251 -> [w274 w297]
                  tunnel: w250 -> [w273 w298]
                  frame 0, Default {
                    n99 = Index Array(array=w274, index=w273) -> (element=w272:string)
                    n100 = Index Array(array=w278, index=w277) -> (element=w276:refnum<vi>)
                    n101 = disable-structure shown="Enabled" {
                      disable-tunnel: w280 -> [w283 w288]
                      disable-tunnel: [w282 w294] -> w279
                      disable-tunnel: w276 -> [w281 w293]
                      disable-tunnel: w275 -> [_ w292]
                      disable-tunnel: w272 -> [_ w290]
                      frame Disabled {
                        n102 = invoke class="VI" method="FP.Open"(reference=w281, error in=w283, "Activate"=TRUE ("Activate?"), "State"=T6."Standard") -> (error out=w282:errorcluster)  [unwired: 1 in, 4 out]
                      }
                      frame Enabled {
                        n103 = call "Main - Event Log (eFGV).vi"("Action"=eFGV_States."Write", "error in"=w288, "Fileid"=w290) -> ("error out"=w289:errorcluster)  [unwired: 5 in, 3 out]
                        n104 = Bundle By Name(cluster=T9 {"RunTest"=refnum, "Name"="", "FileId"="", "Status"=""} ("Data"), "Name"=w292, "RunTest"=w293, "FileId"=w290) -> (w286:T9)
                        n105 = call "Main - Run Test Event (eFGV).vi"("Action"=eFGV_States."Write", "error in"=w289, "Data"=w286) -> ("error out"=w294:errorcluster)  [unwired: 6 in, 2 out]
                      }
                    }
                  }
                  frame -1 {
                    n106 = Index Array(array=w297, index=w298) -> (element=w296:string)
                    n107 = Open VI Reference(vi path=w310, error in (no error)=w309) -> (vi reference=w314:refnum<vi>, error out=w315:errorcluster)  [unwired: 4 in]
                    n108 = invoke class="VI" method="Ctrl Val.Set"(reference=w314, error in=w315, "Control Name"="testname", "Value"=w301) -> (reference out=w316:refnum<vi>, error out=w318:errorcluster)  [unwired: 1 in, 3 out]
                    n109 = invoke class="VI" method="Run VI"(reference=w316, error in=w318, "Wait until done"=FALSE ("Wait Until Done"), "Auto Dispose Ref"=FALSE ("Auto Dispose Reference")) -> (reference out=w317:refnum<vi>, error out=w319:errorcluster)  [unwired: 1 in, 3 out]
                    n110 = disable-structure shown="Enabled" {
                      disable-tunnel: w319 -> [w325 w332]
                      disable-tunnel: w317 -> [w324 w329]
                      disable-tunnel: [w321 w331] -> w307
                      disable-tunnel: [w320 w329] -> w303
                      disable-tunnel: w299 -> [_ w328]
                      disable-tunnel: w296 -> [_ w327]
                      frame Disabled {
                        n111 = invoke class="VI" method="FP.Open"(reference=w324, error in=w325, "Activate"=TRUE ("Activate?"), "State"=T6."Standard") -> (reference out=w320:refnum<vi>, error out=w321:errorcluster)  [unwired: 1 in, 3 out]
                      }
                      frame Enabled {
                        n112 = Bundle By Name(cluster=T9 {"RunTest"=refnum, "Name"="", "FileId"="", "Status"=""} ("Data"), "Name"=w328, "RunTest"=w329, "FileId"=w327) -> (w330:T9)
                        n113 = call "Main - Run Test Event (eFGV).vi"("Action"=eFGV_States."Write", "error in"=w332, "Data"=w330) -> ("error out"=w331:errorcluster)  [unwired: 6 in, 2 out]
                      }
                    }
                    n114 = Build Array (concatenate)(w305, w303) -> (w304:refnum<vi>[])
                    n115 = Build Array (concatenate)(w302, w301) -> (w300:string[])
                    n116 = call "Runtest - Deamon Ref (FGV).vi"("Action"=FGV_States."Write", "error in"=w307, "Name"=w300, "Ref in"=w304) -> ("error out"=w306:errorcluster)  [unwired: 5 in, 2 out]
                  }
                }
              }
              frame True {
                n117 = Unbundle By Name(w356) -> ("testname"=w336:string[], "Selected Tag"=w338:string, "NameRun"=w341:string[], "TestNameRun"=w342:string[], "fileid"=w335:string[])
                n118 = Build Path(base path=w350, name or relative path="Modules") -> (appended path=w355:path)
                n119 = Search 1D Array(1D array=w342, element=w338) -> (index of element=w343:i32)  [unwired: 1 in]
                n120 = Match Pattern(string=w338, regular expression="_") -> (before substring=w337:string)  [unwired: 1 in, 3 out]
                n121 = Build Path(base path=w355, name or relative path="Modules - Run Test with Config Load.vit") -> (appended path=w351:path)
                n122 = call "Runtest - Deamon Ref (FGV).vi"("Action"=FGV_States."Read", "error in"=w347) -> ("error out"=w348:errorcluster, "Name out"=w344:string[], "Ref out"=w345:refnum<vi>[])  [unwired: 7 in]
                n123 = Index Array(array=w341, index=w343) -> (element=w340:string)
                n124 = Search 1D Array(1D array=w336, element=w337) -> (index of element=w334:i32)  [unwired: 1 in]
                n125 = Search 1D Array(1D array=w344, element=w338) -> (index of element=w346:i32)  [unwired: 1 in]
                n126 = case shown="0, Default" w346 {
                  selector: w346 -> [w362 _]
                  tunnel: [w364 w389] -> w352
                  tunnel: w351 -> [_ w393]
                  tunnel: w348 -> [w365 w392]
                  tunnel: w338 -> [_ w385]
                  tunnel: w345 -> [w363 w388]
                  tunnel: w344 -> [_ w386]
                  tunnel: w340 -> [w360 w382]
                  tunnel: w335 -> [w359 w381]
                  tunnel: w334 -> [w358 w380]
                  frame 0, Default {
                    n127 = Index Array(array=w359, index=w358) -> (element=w357:string)
                    n128 = Index Array(array=w363, index=w362) -> (element=w361:refnum<vi>)
                    n129 = disable-structure shown="Enabled" {
                      disable-tunnel: w365 -> [w368 w377]
                      disable-tunnel: [w367 w376] -> w364
                      disable-tunnel: w361 -> [w366 w375]
                      disable-tunnel: w360 -> [_ w374]
                      disable-tunnel: w357 -> [_ w372]
                      frame Disabled {
                        n130 = invoke class="VI" method="FP.Open"(reference=w366, error in=w368, "Activate"=TRUE ("Activate?"), "State"=T6."Standard") -> (error out=w367:errorcluster)  [unwired: 1 in, 4 out]
                      }
                      frame Enabled {
                        n131 = Bundle By Name(cluster=T9 {"RunTest"=refnum, "Name"="", "FileId"="", "Status"=""} ("Data"), "Name"=w374, "RunTest"=w375, "FileId"=w372) -> (w373:T9)
                        n132 = call "Main - Run Test Event (eFGV).vi"("Action"=eFGV_States."Write", "error in"=w377, "Data"=w373) -> ("error out"=w376:errorcluster)  [unwired: 6 in, 2 out]
                      }
                    }
                  }
                  frame -1 {
                    n133 = Index Array(array=w381, index=w380) -> (element=w379:string)
                    n134 = Open VI Reference(vi path=w393, error in (no error)=w392) -> (vi reference=w397:refnum<vi>, error out=w398:errorcluster)  [unwired: 4 in]
                    n135 = invoke class="VI" method="Ctrl Val.Set"(reference=w397, error in=w398, "Control Name"="testname", "Value"=w385) -> (reference out=w399:refnum<vi>, error out=w401:errorcluster)  [unwired: 1 in, 3 out]
                    n136 = invoke class="VI" method="Run VI"(reference=w399, error in=w401, "Wait until done"=FALSE ("Wait Until Done"), "Auto Dispose Ref"=FALSE ("Auto Dispose Reference")) -> (reference out=w400:refnum<vi>, error out=w402:errorcluster)  [unwired: 1 in, 3 out]
                    n137 = disable-structure shown="Enabled" {
                      disable-tunnel: w402 -> [w408 w415]
                      disable-tunnel: w400 -> [w407 w412]
                      disable-tunnel: [w404 w414] -> w390
                      disable-tunnel: [w403 w412] -> w383
                      disable-tunnel: w382 -> [_ w411]
                      disable-tunnel: w379 -> [_ w410]
                      frame Disabled {
                        n138 = invoke class="VI" method="FP.Open"(reference=w407, error in=w408, "Activate"=TRUE ("Activate?"), "State"=T6."Standard") -> (reference out=w403:refnum<vi>, error out=w404:errorcluster)  [unwired: 1 in, 3 out]
                      }
                      frame Enabled {
                        n139 = Bundle By Name(cluster=T9 {"RunTest"=refnum, "Name"="", "FileId"="", "Status"=""} ("Data"), "Name"=w411, "RunTest"=w412, "FileId"=w410) -> (w413:T9)
                        n140 = call "Main - Run Test Event (eFGV).vi"("Action"=eFGV_States."Write", "error in"=w415, "Data"=w413) -> ("error out"=w414:errorcluster)  [unwired: 6 in, 2 out]
                      }
                    }
                    n141 = Build Array (concatenate)(w388, w383) -> (w387:refnum<vi>[])
                    n142 = Build Array (concatenate)(w386, w385) -> (w384:string[])
                    n143 = call "Runtest - Deamon Ref (FGV).vi"("Action"=FGV_States."Write", "error in"=w390, "Name"=w384, "Ref in"=w387) -> ("error out"=w389:errorcluster)  [unwired: 5 in, 2 out]
                  }
                }
              }
            }
          }
          frame "Close" {
            n144 = control-ref of="This VI"() -> (w419:refnum<vi>)
            n145 = invoke class="VI" method="FP.Close"(reference=w419, error in=w418) -> (error out=w417:errorcluster)  [unwired: 1 in, 2 out]
          }
          frame "Exit" {
          }
        }
      }
      frame Error {
        n146 = call <vilib>:"Clear Errors.vi"("error in (no error)"=w433) -> ("error out"=w432:errorcluster)  [unwired: 5 in, 1 out]
        n147 = Wait (ms)(milliseconds to wait=u32 100) -> ()  [unwired: 1 out]
      }
    }
  }
  "error out" <- w8
